vi "system_tdms_write.vi"(7 "Timer in":dbl format="%#_13g", 8 "error in (no error)":errorcluster, 10 "Robot Mode in":T1, 11 "tdms refnum in":refnum<k34>) -> (0 "error out":errorcluster, 2 "Robot Mode out":T1, 3 "tdms refnum out":refnum<k34>)   [LabVIEW 2017, in "labview-standard-library.lvlib"]
uses:
  <vilib>/Rock Robotics/WPI/DriverStation/WPI_DriverStationRobotMode2.ctl
  labview-standard-library.lvlib
panel:
  in  "Testing_code?":bool
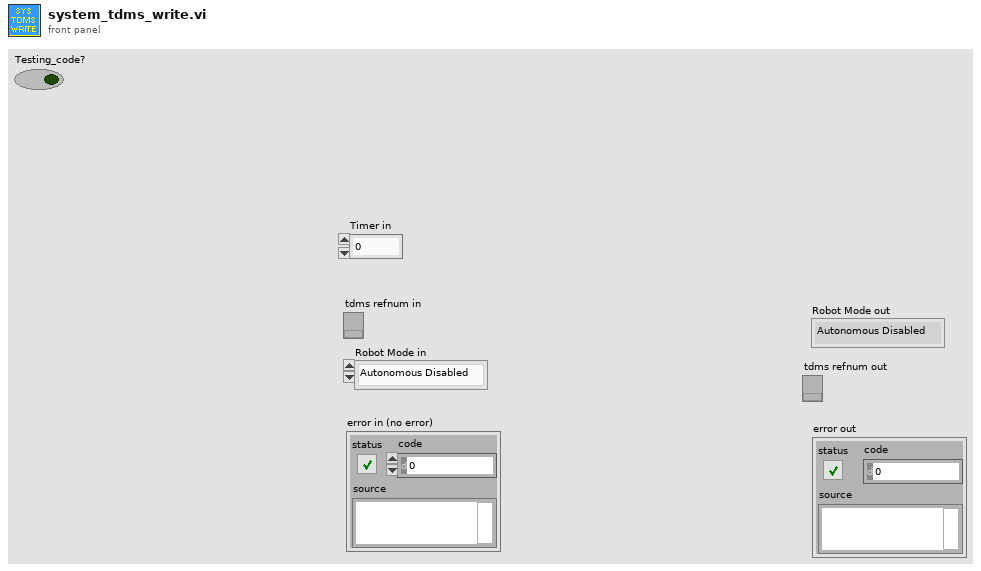
[diagram p1: front panel]
types:
  T1 = typedef "WPI_DriverStationRobotMode2.ctl" = enum16{"Autonomous Disabled", "Autonomous Enabled", "Teleop Disabled", "Teleop Enabled", "Disconnected", "Finish", "Test Disabled", "Test Enabled", "Emergency Stopped"}
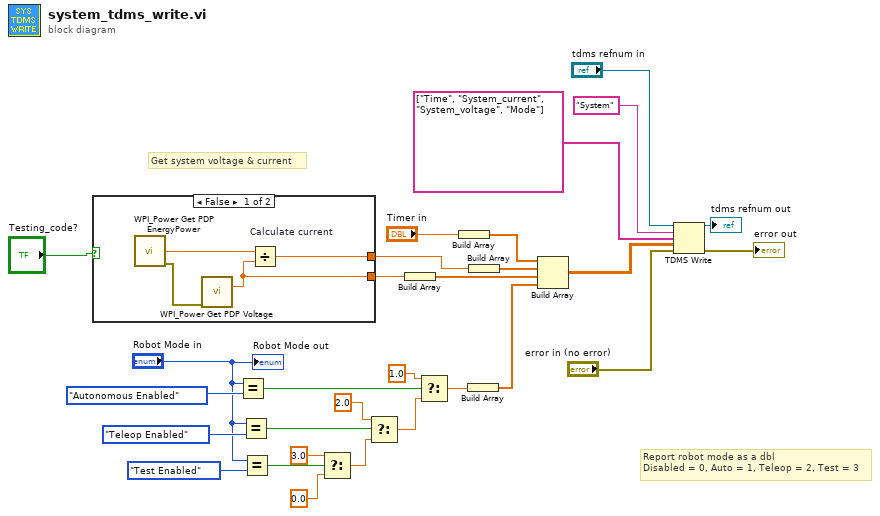
[diagram p0: block diagram]
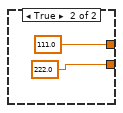
[diagram p2: hidden frame]
diagram:
  # "Get system voltage & current"
  # "Report robot mode as a dbl\nDisabled = 0, Auto = 1, Teleop = 2, Test = 3"
  n1 = case shown="False" "Testing_code?" {
    tunnel: [w32 111.0] -> w17
    tunnel: [w31 222.0] -> w16
    frame False {
      n2 = call <vilib>:"WPI_Power Get PDP EnergyPower.vi"() -> ("Power (W)"=w33:dbl, "error out"=w30:errorcluster)  [unwired: 13 in, 1 out]
      n3 = call <vilib>:"WPI_Power Get PDP Voltage.vi"("error in"=w30) -> ("voltage (V)"=w31:dbl)  [unwired: 13 in, 1 out]
      n4 = Divide "Calculate current"(x=w33, y=w31) -> (x/y=w32:dbl)
    }
    frame True {
    }
  }
  n5 = Equal?(x="Robot Mode in", y=WPI_DriverStationRobotMode2."Autonomous Enabled" ("Robot Mode")) -> (x = y?=w25:bool)
  n6 = Equal?(x="Robot Mode in", y=WPI_DriverStationRobotMode2."Teleop Enabled" ("Robot Mode")) -> (x = y?=w11:bool)
  n7 = Equal?(x="Robot Mode in", y=WPI_DriverStationRobotMode2."Test Enabled") -> (x = y?=w12:bool)
  n8 = Select(t=3.0, s=w12, f=0.0) -> (s? t:f=w10:dbl)
  n9 = Select(t=2.0, s=w11, f=w10) -> (s? t:f=w24:dbl)
  n10 = Build Array(w16) -> (w2:dbl[])
  n11 = Select(t=1.0, s=w25, f=w24) -> (s? t:f=w15:dbl)
  n12 = Build Array("Timer in") -> (w4:dbl[])
  n13 = Build Array(w15) -> (w1:dbl[])
  n14 = Build Array(w17) -> (w3:dbl[])
  n15 = Build Array(w4, w3, w2, w1) -> (w5:dbl[][])
  n16 = TDMS Write(0:"tdms refnum in", 5:"System" ("group name in (Untitled)"), 7:string[] ["Time", "System_current", "System_voltage", "Mode"], 9:w5, 11:"error in (no error)") -> (4:→"tdms refnum out":refnum<k34>, 15:→"error out":errorcluster)  [unwired: 1 in, 2 out]
  "Robot Mode out" <- "Robot Mode in"
